vi "Init.vi"(6 "Channels":T1[](array[typedef]), 8 "error in (no error)":errorcluster, 9 "Raw Values (T)":bool=TRUE, 10 "Publish Config (None)":T2, 11 "Group Info":T3) -> (0 "error out":errorcluster, 3 "Group Config out":refnum<class "Group Config.lvclass">)   [LabVIEW 2020, in "Vecto.lvlib" / "Group Config.lvclass"]
uses:
  Group Config.lvclass
  Group Info.ctl
  Publish Config.ctl
  Channel Init.ctl
  Group Config.lvclass/Group Config.ctl
  Vecto.lvlib
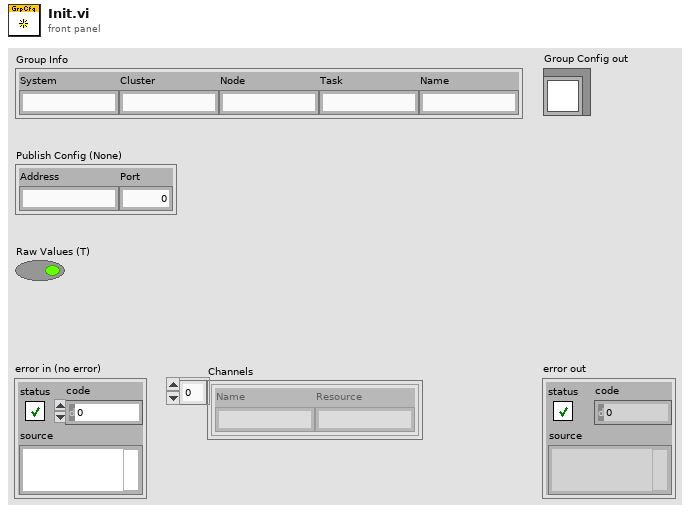
[diagram p1: front panel]
types:
  T1 = typedef "Vecto.lvlib/Channel Init.ctl" = cluster{"Name":string, "Resource":string}
  T2 = typedef "Vecto.lvlib/Publish Config.ctl" = cluster{"Address":string, "Port":u16}
  T3 = typedef "Vecto.lvlib/Group Info.ctl" = cluster{"System":string, "Cluster":string, "Node":string, "Task":string, "Name":string}
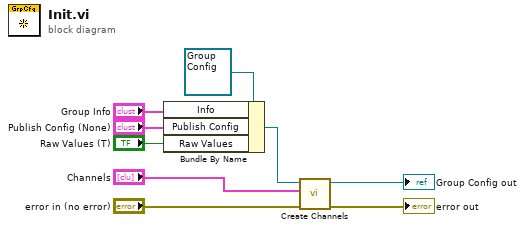
[diagram p0: block diagram]
diagram:
  n1 = Bundle By Name(cluster=refnum<class "Group Config.lvclass"> refnum ("Group Config in"), "Info"="Group Info", "Publish Config"="Publish Config (None)", "Raw Values"="Raw Values (T)") -> (w3:refnum<class "Group Config.lvclass">)
  n2 = call "Create Channels.vi"("error in (no error)"="error in (no error)", "Channels"="Channels", "Group Config in"=w3) -> ("error out"=→"error out":errorcluster, "Group Config out"=→"Group Config out":refnum<class "Group Config.lvclass">)  [unwired: 7 in]
